vi "Power Accuracy Pre-Processing.vi"(6 "Username (\"\")":string, 7 "Fields In":T1[](array[typedef]), 8 "error in (no error)":errorcluster, 10 "Test Configuration (\"\")":string, 11 "Test_ID (\"\")":string) -> (0 "error out":errorcluster, 1 "Files Found?":bool, 2 "New Test Configuration":string, 3 "Dup Test_ID":string, 5 "Fields Out":T1[](array[typedef]))   [LabVIEW 2011]
uses:
  server/database/Fields/Field Record.ctl
  server/database/Fields/Field DataTypes.ctl
  server/database/Fields/Field NextItem.ctl
  LIB/Power Accuracy Version.vi
  Summitek EXT/OpenG EXT/array/array.llb/Remove Duplicates from 1D Array (String)__ogtk.vi
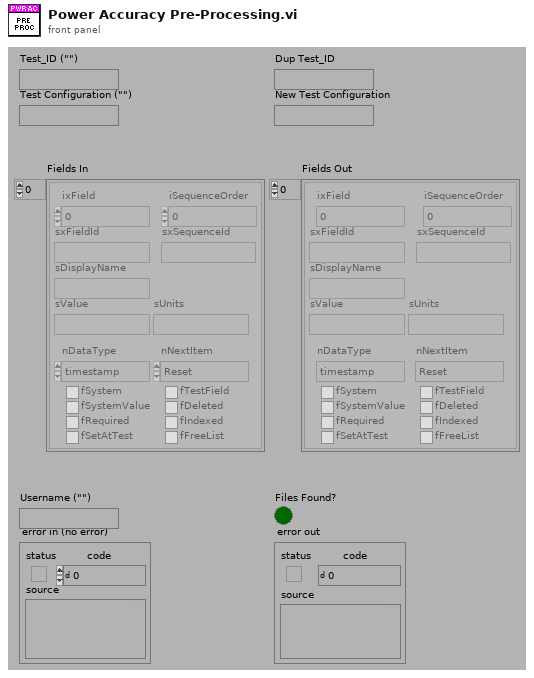
[diagram p1: front panel]
types:
  T1 = typedef "Field Record.ctl" = cluster{"ixField":i32, "iSequenceOrder":i32, "sxFieldId":string, "sxSequenceId":string, "sDisplayName":string, "sValue":string, "sUnits":string, "nDataType":T2, "nNextItem":T3, "fSystem":bool, "fSystemValue":bool, "fRequired":bool, "fSetAtTest":bool, "fTestField":bool, "fDeleted":bool, "fIndexed":bool, "fFreeList":bool}
  T2 = typedef "Field DataTypes.ctl" = enum32{"text", "numeric", "list", "timestamp", "boolean"}
  T3 = typedef "Field NextItem.ctl" = enum32{"Reset", "Retain", "Auto-Increment"}
  T4 = typedef "Power Accuracy Test Parameters.ctl" = cluster{"Stimulus":T5, "Measurement":T6, "Display":T9, "Limit":T10, "Calibration":T11}
  T5 = typedef "Power Accuracy Stimulus Parameters.ctl" = cluster{"Power Start":i32, "Power Stop":i32, "Frequency Type":enum16{"Band Edges", "Custom"}, "Frequency Points":dbl[], "TX 1 Frequency (MHz)":cluster{"Min":dbl, "Max":dbl}, "TX 2 Frequency (MHz)":cluster{"Min":dbl, "Max":dbl}, "RX Frequency (MHz)":cluster{"Min":dbl, "Max":dbl}, "Pad Model Number":string, "Pad Serial Number":string, "Pad Values":dbl[][][]}
  T6 = typedef "Power Accuracy Measurement Parameters.ctl" = cluster{"DUT Port":T7, "Direction":T8}
  T7 = typedef "DUTport.ctl" = enum16{"Port 1", "Port 2"}
  T8 = typedef "MeasMode.ctl" = u16
  T9 = typedef "Power Accuracy Display Parameters.ctl" = cluster{"Power":cluster{"Min":i32, "Max":i32}, "Tolerance":cluster{"Min":dbl, "Max":dbl}}
  T10 = typedef "Power Accuracy Limit Parameters.ctl" = cluster{"Tolerance":dbl}
  T11 = typedef "Power Accuracy Calibration State.ctl" = cluster{"Calibrated?":bool}
  T12 = typedef "Connection Refnum.ctl" = cluster{"Environment Handle":i32, "Connection Handle":i32}
  T13 = typedef "TDMS File.ctl" = cluster{"File Path":path, "Run Data":T14[], "Serial Number":string, "Model Number":string, "Test Type":string}
  T14 = typedef "TDMS Run.ctl" = cluster{"Channel Data":T15[], "Custom Fields":T1[], "Run ID":string}
  T15 = typedef "TDMS Channel (Sxx).ctl" = cluster{"Channel Name":string, "Waveform":dbl[], "Unit":string, "List value":string}
  T16 = typedef "OGAB Version.ctl" = cluster{"Version":string, "Build Number":u32, "Build Date/Time":dbl}
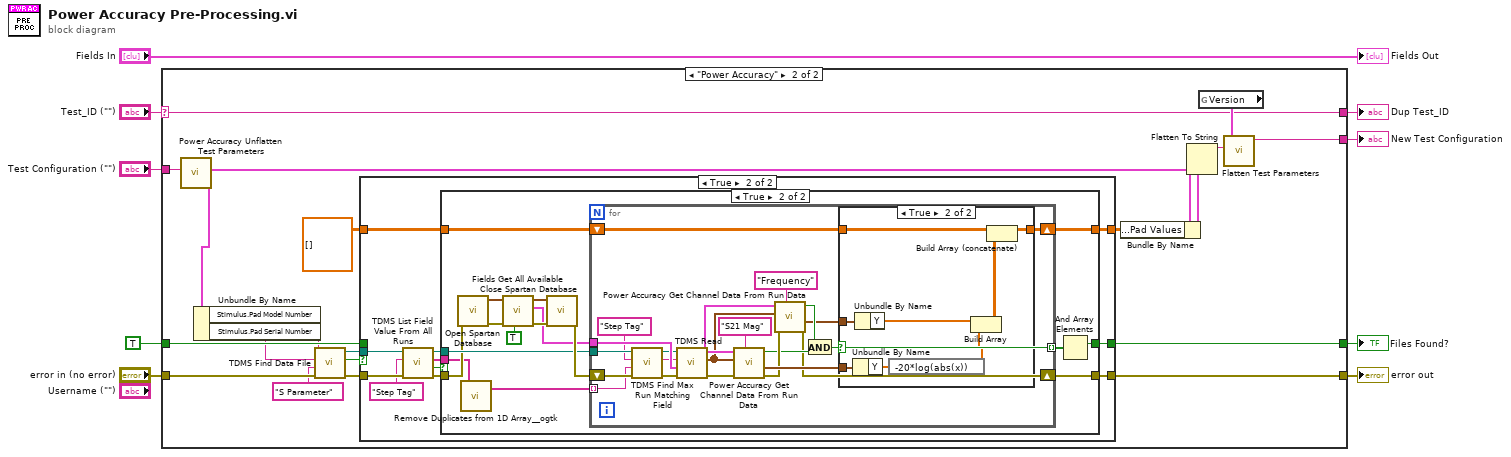
[diagram p0: block diagram]
diagram:
  n1 = case shown="\"Power Accuracy\"" "Test_ID (\"\")" {
    selector: "Test_ID (\"\")" -> [w11 w24]
    tunnel: [w11 w24] -> w9
    tunnel: "Test Configuration (\"\")" -> [w13 w32]
    tunnel: [w13 w28] -> w7
    tunnel: "error in (no error)" -> [w12 w27]
    tunnel: [w12 w26] -> w4
    tunnel: TRUE -> [w10 w23]
    tunnel: [w10 w22] -> w1
    frame Default {
    }
    frame "Power Accuracy" {
      n2 = call "Power Accuracy Unflatten Test Parameters.vi"("Parameter String"=w32) -> ("Power Accuracy Test Parameters"=w25:T4)  [unwired: 8 in, 2 out]
      n3 = Unbundle By Name(w25) -> ("Stimulus.Pad Model Number"=w15:string, "Stimulus.Pad Serial Number"=w14:string)
      n4 = call "TDMS Find Data File.vi"("error in (no error)"=w27, "Test Type"="S Parameter" ("Value"), "Serial Number"=w14, "Model Number"=w15) -> ("error out"=w19:errorcluster, "Found?"=w18:bool, "TDMS Path"=w20:path)  [unwired: 5 in]
      n5 = case shown="True" w18 {
        tunnel: [w34 w41] -> w26
        tunnel: w23 -> [_ _]
        tunnel: [_ w38] -> w22
        tunnel: w20 -> [_ w44]
        tunnel: w19 -> [w34 w45]
        tunnel: [w33 w37] -> w17
        tunnel: dbl[][][] [] ("Stimulus.Pad Values") -> [w33 w36]
        frame False {
          # "No File Found."
        }
        frame True {
          n6 = call "TDMS List Field Value From All Runs.vi"("error in (no error)"=w45, "Property Name"="Step Tag" ("Value"), "TDMS File Path"=w44) -> ("error out"=w40:errorcluster, "Found?"=w35:bool, "Property Values"=w39:string[], "TDMS File Path Out"=w43:path)  [unwired: 5 in]
          n7 = case shown="True" w35 {
            tunnel: w43 -> [_ w56]
            tunnel: [w47 w55] -> w41
            tunnel: w40 -> [w47 w54]
            tunnel: w39 -> [_ w53]
            tunnel: [_ w50] -> w38
            tunnel: [w46 w49] -> w37
            tunnel: w36 -> [w46 w48]
            frame False {
            }
            frame True {
              n8 = call "Open Spartan Database.vi"("error in (no error)"=w54) -> ("error out"=w59:errorcluster, "Connection Refnum"=w60:T12)  [unwired: 9 in]
              n9 = call-poly "Remove Duplicates from 1D Array__ogtk.vi"("Input Array"=w53) -> ("Output Array"=w52:string[])  [unwired: 1 out]
              n10 = call "Fields Get All Available.vi"("Combine All? (f)"=TRUE, "error in (no error)"=w59, "Connection Refnum"=w60) -> ("error out"=w62:errorcluster, "System or ALL Combined Fields"=w57:T1[], "Connection Refnum"=w63:T12)  [unwired: 3 in, 3 out]
              n11 = call "Close Spartan Database.vi"("error in (no error)"=w62, "Connection Refnum"=w63) -> ("error out"=w58:errorcluster)  [unwired: 9 in]
              n12 = for {
                tunnel: w57 -> [w85]
                tunnel: w56 -> [w83]
                tunnel: w52 -> [w79] mode=indexing
                shift-right: [w67] -> w55
                shift-left: w58 -> [w84]
                shift-right: [w66] -> w49
                shift-left: w48 -> [w68]
                tunnel: [w65] -> w51 mode=indexing
                n13 = call "TDMS Find Max Run Matching Field.vi"("error in (no error)"=w84, "Property Value"=w79, "Property Name"="Step Tag" ("Value"), "TDMS File Path"=w83) -> ("error out"=w81:errorcluster, "Run ID"=w64:string, "TDMS File Path Out"=w82:path)  [unwired: 4 in, 1 out]
                n14 = call "TDMS Read.vi"("error in (no error)"=w81, "System or ALL Combined Fields"=w85, "Run String"=w64, "TDM File Path"=w82) -> ("error out"=w78:errorcluster, "Run Waveforms"=w70:waveform(dbl)[], "File Information"=w71:T13)  [unwired: 3 in, 2 out]
                n15 = call "Power Accuracy Get Channel Data From Run Data.vi"("Channel Name"="S21 Mag" ("Value"), "error in (no error)"=w78, "Run Waveforms"=w70, "File Information"=w71) -> ("error out"=w74:errorcluster, "Data Waveform"=w77:waveform(dbl), "Found?"=w72:bool)  [unwired: 5 in]
                n16 = call "Power Accuracy Get Channel Data From Run Data.vi"("Channel Name"="Frequency" ("Value"), "error in (no error)"=w74, "Run Waveforms"=w70, "File Information"=w71) -> ("error out"=w67:errorcluster, "Data Waveform"=w69:waveform(dbl), "Found?"=w73:bool)  [unwired: 5 in]
                n17 = And(x=w73, y=w72) -> (x .and. y?=w65:bool)
                n18 = case shown="True" w65 {
                  tunnel: w77 -> [_ w94]
                  tunnel: w69 -> [_ w93]
                  tunnel: w68 -> [w86 w92]
                  tunnel: [w86 w87] -> w66
                  frame False {
                  }
                  frame True {
                    n19 = Unbundle By Name(w94) -> ("Y"=w89:dbl[])
                    n20 = Unbundle By Name(w93) -> ("Y"=w91:dbl[])
                    n21 = expression code="-20*log(abs(x))"(w89) -> (w88:dbl[])
                    n22 = Build Array(w91, w88) -> (w90:dbl[][])
                    n23 = Build Array (concatenate)(w92, w90) -> (w87:dbl[][][])
                  }
                }
              }
              n24 = And Array Elements(Boolean array=w51) -> (logical AND=w50:bool)
            }
          }
        }
      }
      n25 = Bundle By Name(cluster=w25, "Stimulus.Pad Values"=w17) -> (w29:T4)
      n26 = Flatten To String(anything=w29) -> (data string=w31:string)  [unwired: 1 in, 4 out]
      n27 = global read "Power Accuracy Version.vi" "Version"() -> (w30:T16)
      n28 = call "Flatten Test Parameters.vi"("Flattened Test Parameters (\"\")"=w31, "Test Version"=w30) -> ("Flattened Test Parameters with Version"=w28:string)  [unwired: 1 in, 4 out]
    }
  }
  "error out" <- w4
  "New Test Configuration" <- w7
  "Dup Test_ID" <- w9
  "Files Found?" <- w1
  "Fields Out" <- "Fields In"
